vi "Init from INI File.vi"(8 "error in (no error)":errorcluster, 10 "ini file":path, 11 "CS++GoBangClient in":refnum<class "CS++GoBangClient.lvclass">) -> (0 "error out":errorcluster, 3 "CS++GoBangClient out":refnum<class "CS++GoBangClient.lvclass">)   [LabVIEW 2014, in "GoBang.lvlib" / "CS++GoBangClient.lvclass"]
uses:
  CS++GoBangClient.lvclass
  CS++GoBangClient.lvclass/CS++GoBangClient.ctl
  <vilib>/Utility/config.llb/Read Key (String).vi
  <vilib>/Utility/config.llb/NI_LVConfig.lvlib
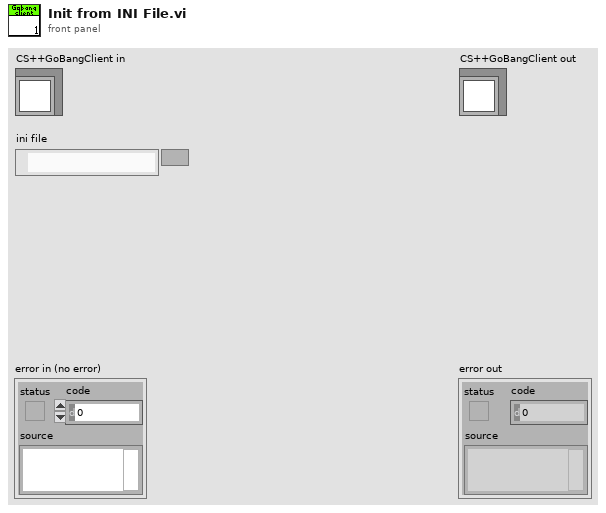
[diagram p1: front panel]
types:
  T1 = typedef "NI_LVConfig.lvlib/Config Data RefNum.ctl" = refnum<k1>
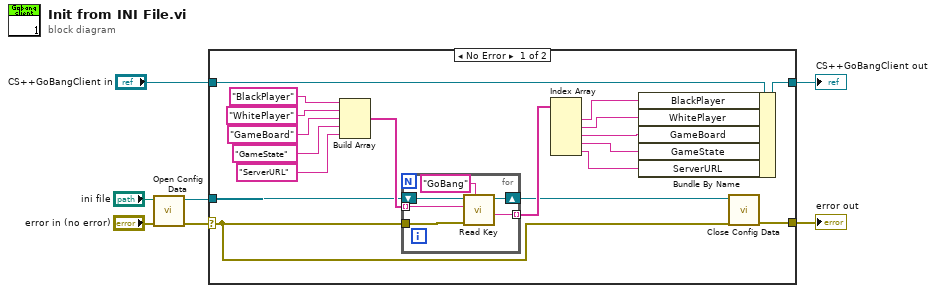
[diagram p0: block diagram]
diagram:
  n1 = call <vilib>:"Open Config Data.vi"("error in (no error)"="error in (no error)", "configuration file path"="ini file") -> ("error out"=w3:errorcluster, "refnum"=w1:T1)  [unwired: 7 in, 1 out]
  n2 = case shown="No Error" w3 {
    selector: w3 -> [w8 w33]
    tunnel: [w10 w33] -> w7
    tunnel: [w24 w32] -> w5
    tunnel: "CS++GoBangClient in" -> [w25 w32]
    tunnel: w1 -> [w17 _]
    frame No Error {
      n3 = Build Array("BlackPlayer" ("name"), "WhitePlayer", "GameBoard", "GameState", "ServerURL") -> (w18:string[])
      n4 = for {
        tunnel: w8 -> [w31]
        tunnel: w18 -> [w30] mode=indexing
        tunnel: [w27] -> w16 mode=indexing
        shift-right: [w26] -> w9
        shift-left: w17 -> [w29]
        n5 = call-poly <vilib>:"Read Key.vi"("section"="GoBang", "error in (no error)"=w31, "key"=w30, "refnum"=w29) -> ("value"=w27:string, "refnum out"=w26:T1)  [unwired: 4 in, 2 out]
      }
      n6 = Index Array(array=w16) -> (element #1=w15:string, element #2=w14:string, element #3=w13:string, element #4=w12:string, element #5=w11:string)  [unwired: 5 in]
      n7 = Bundle By Name(cluster=w25, "BlackPlayer"=w15, "WhitePlayer"=w14, "GameBoard"=w13, "GameState"=w12, "ServerURL"=w11) -> (w24:refnum<class "CS++GoBangClient.lvclass">)
      n8 = call <vilib>:"Close Config Data.vi"("error in (no error)"=w8, "refnum"=w9) -> ("error out"=w10:errorcluster)  [unwired: 8 in, 1 out]
    }
    frame Error {
    }
  }
  "error out" <- w7
  "CS++GoBangClient out" <- w5
